vi "ArmCurlSystem.vi"(10 "Secondary Joystick Buttons":bool[](array[boolean]), 11 "Secondary Joystick Values":dbl[](array[numeric])) -> ()   [LabVIEW 2018]
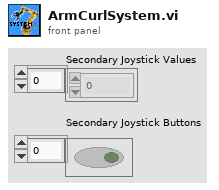
[diagram p1: front panel]
types:
  T1 = typedef "SecondaryJoystickButtons.ctl" = cluster{"Intake":bool, "Outtake":bool, "ShoulderMotor":bool, "ElbowMotor":bool, "Open Grip":bool, "Close Grip":bool}
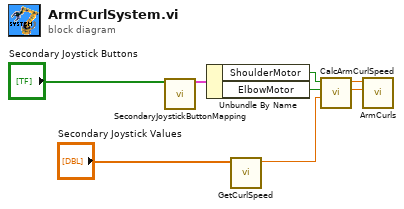
[diagram p0: block diagram]
diagram:
  n1 = call "SecondaryJoystickButtonMapping.vi"("Secondary joystick buttons"="Secondary Joystick Buttons") -> ("SecondaryJoystickButtons"=w3:T1)  [unwired: 13 in, 1 out]
  n2 = Unbundle By Name(w3) -> ("ShoulderMotor"=w1:bool, "ElbowMotor"=w2:bool)
  n3 = call "GetCurlSpeed.vi"("SecondaryJoystickValues"="Secondary Joystick Values") -> ("Curl Speed"=w5:dbl)  [unwired: 10 in]
  n4 = call "CalcArmCurlSpeed.vi"("Curl Speed"=w5, "Elbow Motor"=w2, "Shoulder Motor"=w1) -> ("Elbow Speed"=w6:dbl, "Shoulder Speed"=w7:dbl)  [unwired: 7 in]
  n5 = call "ArmCurls.vi"("Elbow Speed"=w6, "shoulder speed"=w7) -> ()  [unwired: 10 in]
